vi "Read Shared Library.vi"(8 "Error In":errorcluster, 11 "SSH In":refnum<class "SSH.lvclass">) -> (0 "Error Out":errorcluster, 2 "lv-libssh2 Shared Library":path, 3 "SSH Out":refnum<class "SSH.lvclass">)   [LabVIEW 2018, in "Toolkit.lvlib" / "SSH.lvclass"]
uses:
  SSH.lvclass
  SSH.lvclass/SSH.ctl
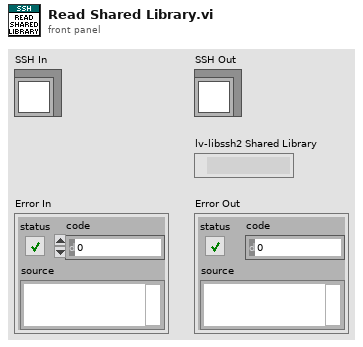
[diagram p1: front panel]
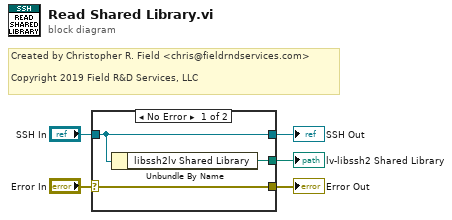
[diagram p0: block diagram]
diagram:
  # "Created by Christopher R. Field <chris@fieldrndservices.com>\n\nCopyright 2019 Field R&D Services, LLC"
  n1 = case shown="No Error" "Error In" {
    selector: "Error In" -> [w6 w9]
    tunnel: "SSH In" -> [w8 w10]
    tunnel: [w8 w10] -> w3
    tunnel: [w7 _] -> w2
    tunnel: [w6 w9] -> w1
    frame No Error {
      n2 = Unbundle By Name(w8) -> ("libssh2lv Shared Library"=w7:path)
    }
    frame Error {
    }
  }
  "SSH Out" <- w3
  "lv-libssh2 Shared Library" <- w2
  "Error Out" <- w1
